vi "Engine Out - Diesel - Boost Actuation.vi"(10 "Wastegate1 Position (%Open)":sgl, 11 "VGT1 Position (%Open)":sgl) -> (2 "Wastegate LS Output":T1, 3 "VGT LS Output":T1)   [LabVIEW 2015, in "ECS-RT.lvlib"]
uses:
  ECS-RT.lvlib
  Typedefs/Raw Outputs/LS.ctl
  ECS-Shared.lvlib
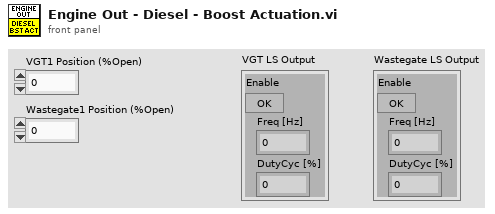
[diagram p1: front panel]
types:
  T1 = typedef "ECS-Shared.lvlib/LS.ctl" = cluster{"Enable":bool, "Freq [Hz]":sgl, "DutyCyc [%]":sgl}
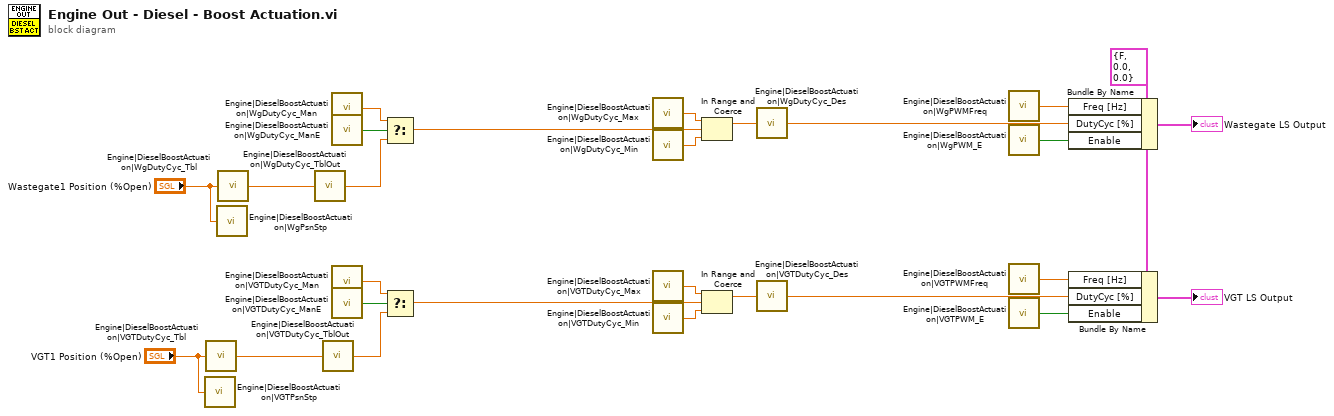
[diagram p0: block diagram]
diagram:
  w9 = T1 {"Enable"=FALSE, "Freq [Hz]"=0.0, "DutyCyc [%]"=0.0} ("LS Output")
  n1 = call "Engine|DieselBoostActuation|VGTPsnStp"("Value"="VGT1 Position (%Open)") -> ()
  n2 = call "Engine|DieselBoostActuation|VGTDutyCyc_Tbl"("X Index"="VGT1 Position (%Open)") -> ("Y"=w4:sgl)
  n3 = call "Engine|DieselBoostActuation|WgPsnStp"("Value"="Wastegate1 Position (%Open)") -> ()
  n4 = call "Engine|DieselBoostActuation|WgDutyCyc_Tbl"("X Index"="Wastegate1 Position (%Open)") -> ("Y"=w3:sgl)
  n5 = call "Engine|DieselBoostActuation|WgDutyCyc_TblOut"("Value"=w3) -> ()
  n6 = call "Engine|DieselBoostActuation|VGTDutyCyc_TblOut"("Value"=w4) -> ()
  n7 = call "Engine|DieselBoostActuation|WgDutyCyc_Man"() -> ("Value"=w13:sgl)
  n8 = call "Engine|DieselBoostActuation|WgDutyCyc_ManE"() -> ("Value"=w14:bool)
  n9 = call "Engine|DieselBoostActuation|VGTDutyCyc_Man"() -> ("Value"=w12:sgl)
  n10 = call "Engine|DieselBoostActuation|VGTDutyCyc_ManE"() -> ("Value"=w11:bool)
  n11 = Select(t=w13, s=w14, f=w3) -> (s? t:f=w15:sgl)
  n12 = Select(t=w12, s=w11, f=w4) -> (s? t:f=w10:sgl)
  n13 = call "Engine|DieselBoostActuation|WgDutyCyc_Max"() -> ("Value"=w16:sgl)
  n14 = call "Engine|DieselBoostActuation|WgDutyCyc_Min"() -> ("Value"=w17:sgl)
  n15 = call "Engine|DieselBoostActuation|VGTDutyCyc_Max"() -> ("Value"=w18:sgl)
  n16 = call "Engine|DieselBoostActuation|VGTDutyCyc_Min"() -> ("Value"=w19:sgl)
  n17 = In Range and Coerce(upper limit=w16, x=w15, lower limit=w17) -> (coerced(x)=w2:sgl)  [unwired: 1 out]
  n18 = In Range and Coerce(upper limit=w18, x=w10, lower limit=w19) -> (coerced(x)=w1:sgl)  [unwired: 1 out]
  n19 = call "Engine|DieselBoostActuation|WgDutyCyc_Des"("Value"=w2) -> ()
  n20 = call "Engine|DieselBoostActuation|VGTDutyCyc_Des"("Value"=w1) -> ()
  n21 = call "Engine|DieselBoostActuation|WgPWMFreq"() -> ("Value"=w22:sgl)
  n22 = call "Engine|DieselBoostActuation|WgPWM_E"() -> ("Value"=w21:bool)
  n23 = call "Engine|DieselBoostActuation|VGTPWMFreq"() -> ("Value"=w23:sgl)
  n24 = call "Engine|DieselBoostActuation|VGTPWM_E"() -> ("Value"=w20:bool)
  n25 = Bundle By Name(cluster=w9, "Freq [Hz]"=w22, "DutyCyc [%]"=w2, "Enable"=w21) -> (→"Wastegate LS Output":T1)
  n26 = Bundle By Name(cluster=w9, "Freq [Hz]"=w23, "DutyCyc [%]"=w1, "Enable"=w20) -> (→"VGT LS Output":T1)
